vi "PicoScopeospaAdvancedTriggerPWQ.vi"(0 "handle in":i16=16384, 1 "Pulse Width Qualifier Settings":T3 {"Pulse Width Type" items=["None", "Less Than", "Greater Than", "In Range", "Out of Range"]}, 2 "Pulse Width Qualifier Trigger Properties":T1={"Channel A Trigger Properties"={"Threshold Mode"=0, "Available"=TRUE, "Direction"=2}, "Channel B Trigger Properties"={"Threshold Mode"=0, "Available"=FALSE, "Direction"=2}, "Channel C Trigger Properties"={"Threshold Mode"=0, "Available"=FALSE, "Direction"=2}, "Channel D Trigger Properties"={"Threshold Mode"=0, "Available"=FALSE, "Direction"=2}, "Channel E Trigger Properties"={"Threshold Mode"=0, "Available"=FALSE, "Direction"=2}, "Channel F Trigger Properties"={"Threshold Mode"=0, "Available"=FALSE, "Direction"=2}, "Channel G Trigger Properties"={"Threshold Mode"=0, "Available"=FALSE, "Direction"=2}, "Channel H Trigger Properties"={"Threshold Mode"=0, "Available"=FALSE, "Direction"=2}, "Port 0 Trigger Properties"={"Threshold Mode"=0, "Available"=FALSE, "Direction"=2}, "Port 1 Trigger Properties"={"Threshold Mode"=0, "Available"=FALSE, "Direction"=2}} {"Port 1 Trigger Properties"."Direction" items=["Rising"=2, "Falling"=3, "Rising Lower"=7, "Above"=0, "Below"=1, "Rising or Falling"=4, "Falling Lower"=8, "Below Lower"=6, "Above Lower"=5]; "Port 1 Trigger Properties"."Threshold Mode" items=["Level", "Window"]; "Port 0 Trigger Properties"."Direction" items=["Rising"=2, "Falling"=3, "Rising Lower"=7, "Above"=0, "Below"=1, "Rising or Falling"=4, "Falling Lower"=8, "Below Lower"=6, "Above Lower"=5]; "Port 0 Trigger Properties"."Threshold Mode" items=["Level", "Window"]; "Channel H Trigger Properties"."Direction" items=["Rising"=2, "Falling"=3, "Rising Lower"=7, "Above"=0, "Below"=1, "Rising or Falling"=4, "Falling Lower"=8, "Below Lower"=6, "Above Lower"=5]; "Channel H Trigger Properties"."Threshold Mode" items=["Level", "Window"]; "Channel G Trigger Properties"."Direction" items=["Rising"=2, "Falling"=3, "Rising Lower"=7, "Above"=0, "Below"=1, "Rising or Falling"=4, "Falling Lower"=8, "Below Lower"=6, "Above Lower"=5]; "Channel G Trigger Properties"."Threshold Mode" items=["Level", "Window"]; "Channel F Trigger Properties"."Direction" items=["Rising"=2, "Falling"=3, "Rising Lower"=7, "Above"=0, "Below"=1, "Rising or Falling"=4, "Falling Lower"=8, "Below Lower"=6, "Above Lower"=5]; "Channel F Trigger Properties"."Threshold Mode" items=["Level", "Window"]; "Channel E Trigger Properties"."Direction" items=["Rising"=2, "Falling"=3, "Rising Lower"=7, "Above"=0, "Below"=1, "Rising or Falling"=4, "Falling Lower"=8, "Below Lower"=6, "Above Lower"=5]; "Channel E Trigger Properties"."Threshold Mode" items=["Level", "Window"]; "Channel D Trigger Properties"."Direction" items=["Rising"=2, "Falling"=3, "Rising Lower"=7, "Above"=0, "Below"=1, "Rising or Falling"=4, "Falling Lower"=8, "Below Lower"=6, "Above Lower"=5]; "Channel D Trigger Properties"."Threshold Mode" items=["Level", "Window"]; "Channel C Trigger Properties"."Direction" items=["Rising"=2, "Falling"=3, "Rising Lower"=7, "Above"=0, "Below"=1, "Rising or Falling"=4, "Falling Lower"=8, "Below Lower"=6, "Above Lower"=5]; "Channel C Trigger Properties"."Threshold Mode" items=["Level", "Window"]; "Channel B Trigger Properties"."Direction" items=["Rising"=2, "Falling"=3, "Rising Lower"=7, "Above"=0, "Below"=1, "Rising or Falling"=4, "Falling Lower"=8, "Below Lower"=6, "Above Lower"=5]; "Channel B Trigger Properties"."Threshold Mode" items=["Level", "Window"]; "Channel A Trigger Properties"."Direction" items=["Rising"=2, "Falling"=3, "Rising Lower"=7, "Above"=0, "Below"=1, "Rising or Falling"=4, "Falling Lower"=8, "Below Lower"=6, "Above Lower"=5]; "Channel A Trigger Properties"."Threshold Mode" items=["Level", "Window"]}, 11 "error in":errorcluster, 13 "Pulse Width Qualifier Conditions":T2 {"Port 1" items=["Don't Care", "True", "False"]; "Channel H" items=["Don't Care", "True", "False"]; "Channel G" items=["Don't Care", "True", "False"]; "Channel F" items=["Don't Care", "True", "False"]; "Channel E" items=["Don't Care", "True", "False"]; "Aux" items=["Don't Care", "True", "False"]; "Port 0" items=["Don't Care", "True", "False"]; "Channel D" items=["Don't Care", "True", "False"]; "Channel C" items=["Don't Care", "True", "False"]; "Channel B" items=["Don't Care", "True", "False"]; "Channel A" items=["Don't Care", "True", "False"]; "Condition Logic" items=["AND", "OR", "XOR"]}) -> (4 "handle out":i16=16384, 15 "error out":errorcluster)   [LabVIEW 2010]
doc: "This sub VI is an interface for the advanced trigger features of the oscilloscope to support Pulse width qualifier (PWQ)."
uses:
  ps6000a.dll
  psospa.dll
panel:
  in  "PWQ Info Action XOR":bool=TRUE
  in  "PWQ Info Action OR":bool=TRUE
  # "For Condition Logic Suggested settings;\nFor AND, XOR logic-(parallel triggers)\nUse level-type triggers (Level or Inside/outside Window Triggers)\n\nFor OR logic- (single channel)\nUse edge types (e.g. rising, falling, entering window)"
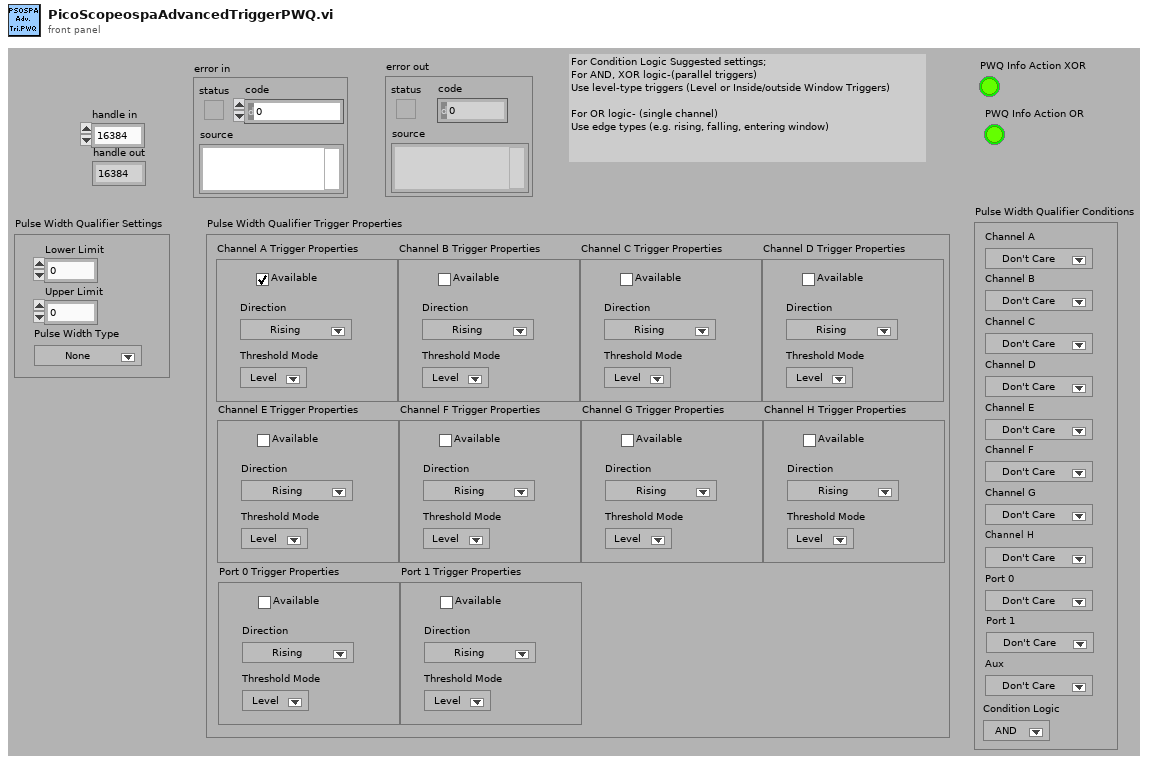
[diagram p1: front panel]
types:
  T1 = cluster{"Channel A Trigger Properties":cluster{"Threshold Mode":i32, "Available":bool, "Direction":u32}, "Channel B Trigger Properties":cluster{"Threshold Mode":i32, "Available":bool, "Direction":u32}, "Channel C Trigger Properties":cluster{"Threshold Mode":i32, "Available":bool, "Direction":u32}, "Channel D Trigger Properties":cluster{"Threshold Mode":i32, "Available":bool, "Direction":u32}, "Channel E Trigger Properties":cluster{"Threshold Mode":i32, "Available":bool, "Direction":u32}, "Channel F Trigger Properties":cluster{"Threshold Mode":i32, "Available":bool, "Direction":u32}, "Channel G Trigger Properties":cluster{"Threshold Mode":i32, "Available":bool, "Direction":u32}, "Channel H Trigger Properties":cluster{"Threshold Mode":i32, "Available":bool, "Direction":u32}, "Port 0 Trigger Properties":cluster{"Threshold Mode":i32, "Available":bool, "Direction":u32}, "Port 1 Trigger Properties":cluster{"Threshold Mode":i32, "Available":bool, "Direction":u32}}
  T2 = cluster{"Channel A":u16, "Channel B":u16, "Channel C":u16, "Channel D":u16, "Channel E":u16, "Channel F":u16, "Channel G":u16, "Channel H":u16, "Port 0":u16, "Port 1":u16, "Aux":u16, "Condition Logic":u16}
  T3 = cluster{"Lower Limit":u32, "Upper Limit":u32, "Pulse Width Type":u32}
  T4 = cluster{"Threshold Mode":i32, "Available":bool, "Direction":u32}[]
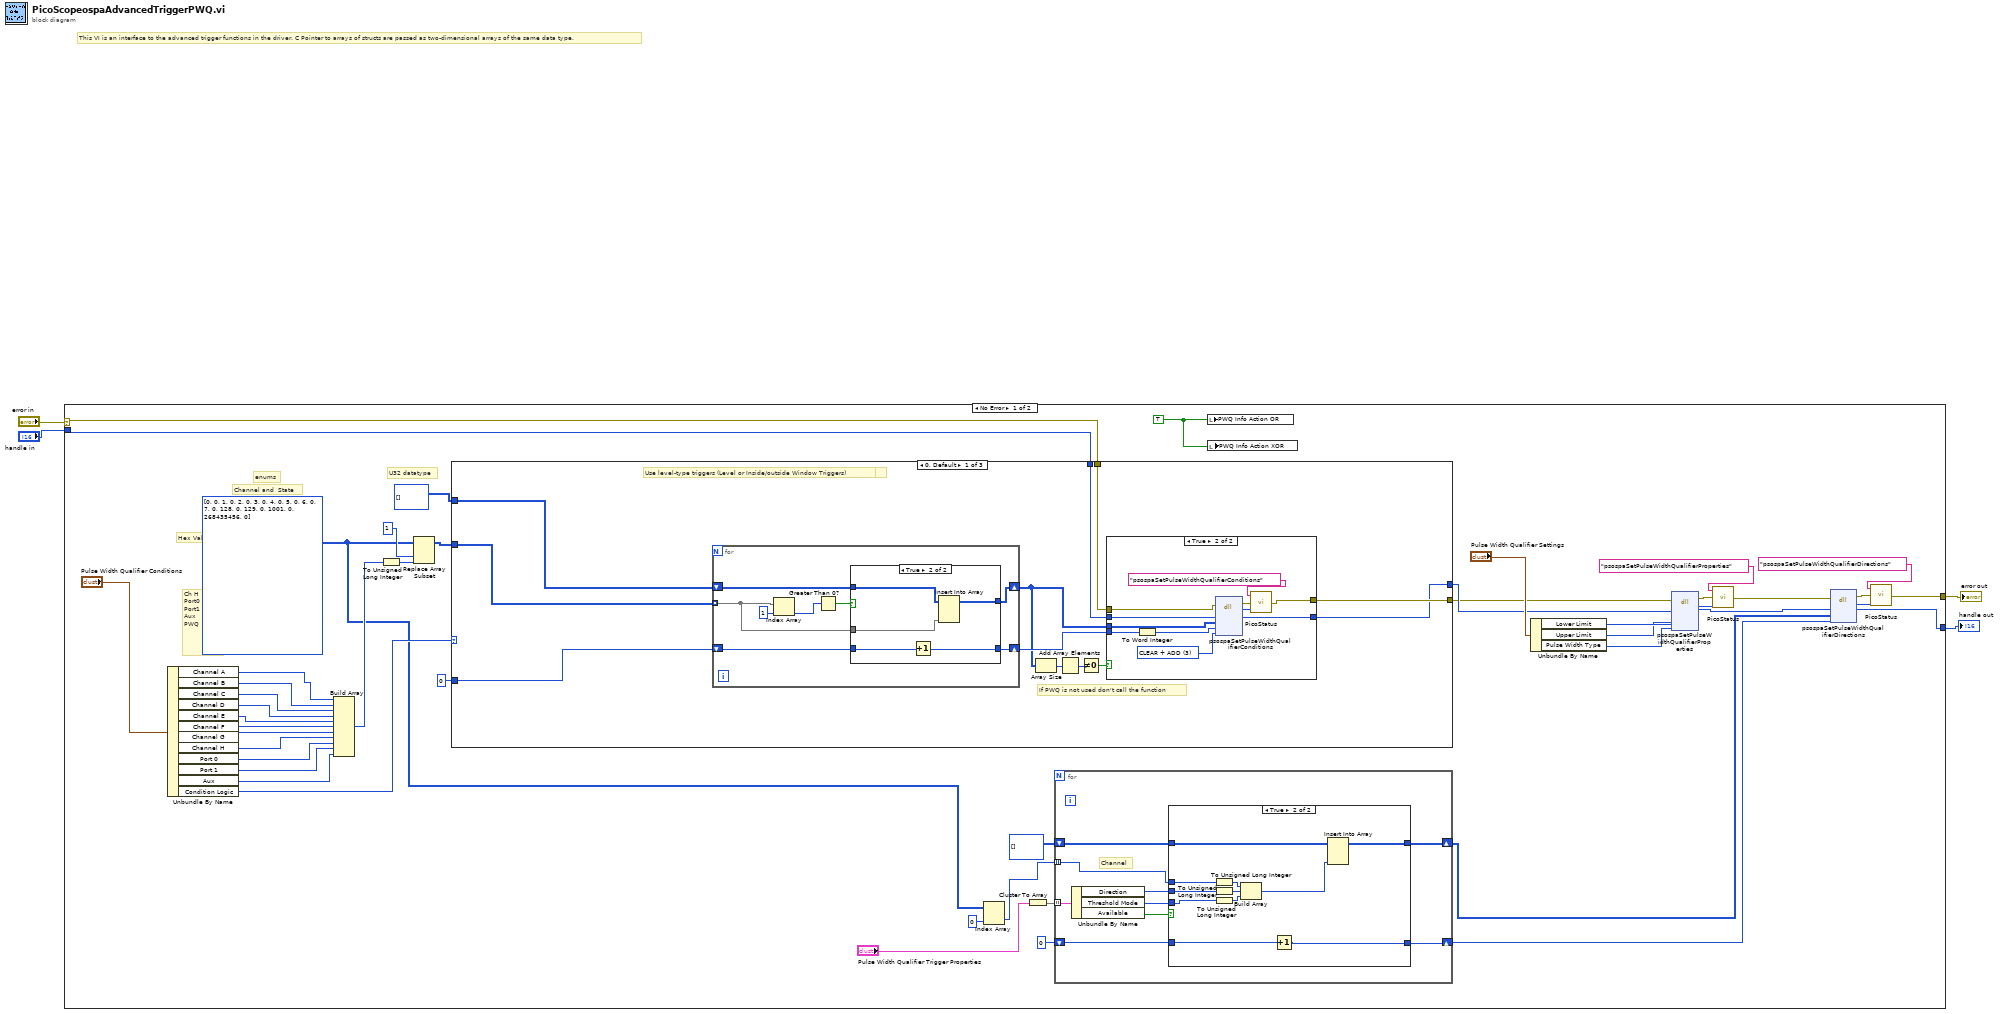
[diagram p0: block diagram]
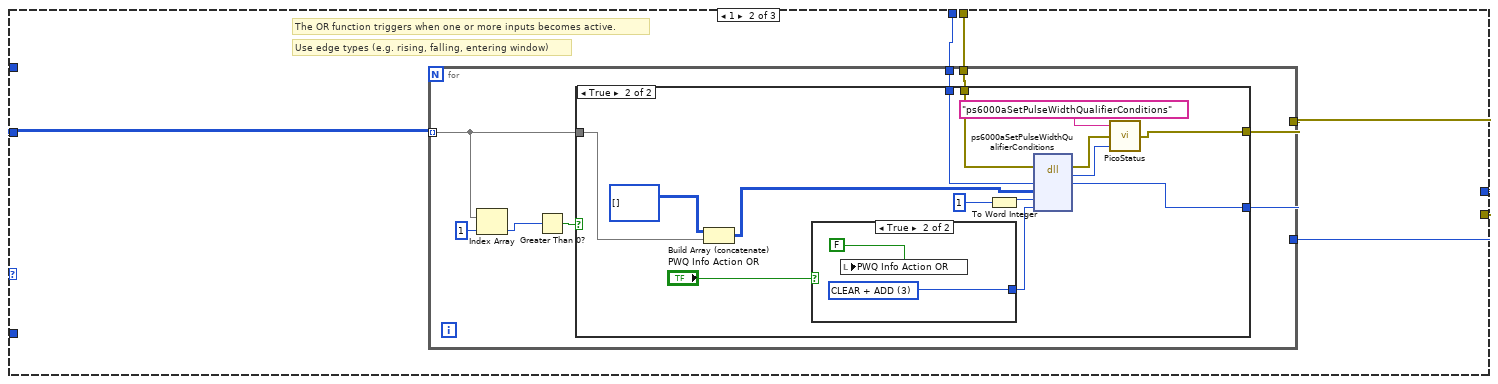
[diagram p5: hidden frame]
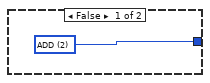
[diagram p7: hidden frame]
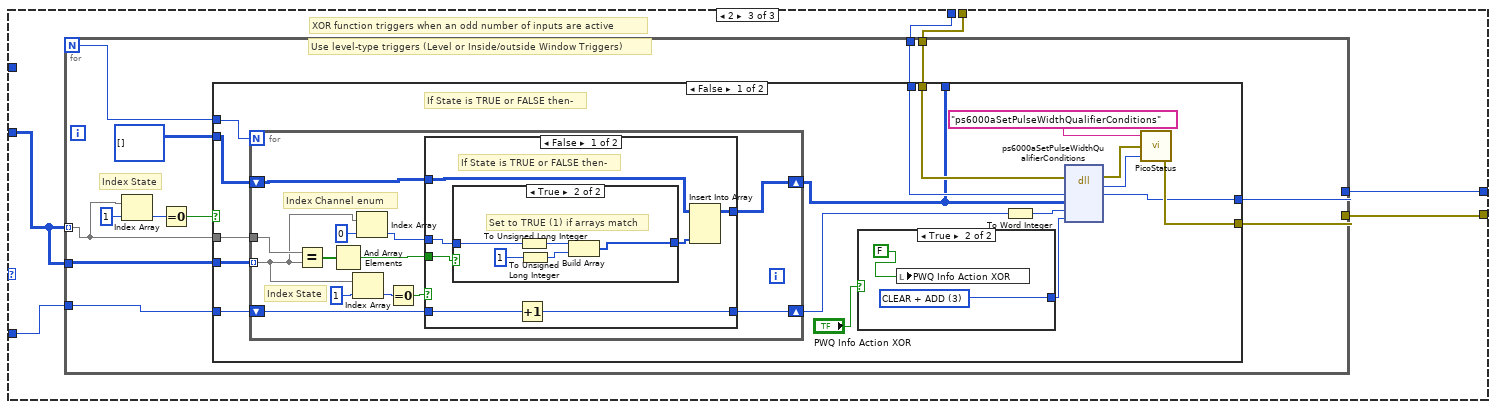
[diagram p8: hidden frame]
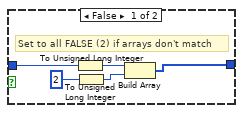
[diagram p9: hidden frame]
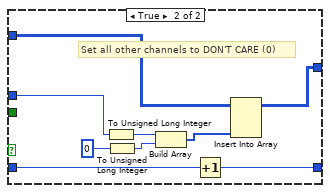
[diagram p10: hidden frame]
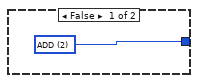
[diagram p11: hidden frame]
diagram:
  # "This VI is an interface to the advanced trigger functions in the driver. C Pointer to arrays of structs are passed as two-dimensional arrays of the same data type."
  n1 = case shown="No Error" "error in" {
    selector: "error in" -> [w6 w226]
    tunnel: "handle in" -> [w5 w227]
    tunnel: [w7 w227] -> w2
    tunnel: [w8 w226] -> w1
    frame No Error {
      w26 = TRUE ("PWQ Info Action XOR")
      w9 = u32[][] [[0, 0], [1, 0], [2, 0], [3, 0], [4, 0], [5, 0], [6, 0], [7, 0], [128, 0], [129, 0], [1001, 0], [268435456, 0]]
      # "U32 datatype"
      # "enums"
      # "Ch H\nPort0\nPort1\nAux\nPWQ"
      # "Channel and  State"
      # "Hex Values"
      n2 = Unbundle By Name("Pulse Width Qualifier Conditions") -> ("Channel A"=w36:u16, "Channel B"=w35:u16, "Channel C"=w34:u16, "Channel D"=w33:u16, "Channel E"=w32:u16, "Channel F"=w31:u16, "Channel G"=w30:u16, "Channel H"=w29:u16, "Port 0"=w28:u16, "Port 1"=w27:u16, "Aux"=w10:u16, "Condition Logic"=w11:u16)
      n3 = Build Array(w36, w35, w34, w33, w32, w31, w30, w29, w28, w27, w10) -> (w50:u16[])
      n4 = To Unsigned Long Integer(number=w50) -> (unsigned 32bit integer=w39:u32[])
      n5 = Replace Array Subset(array=w9, new element=w39, index (col)=1 ("disabled index (col)")) -> (w38:u32[][])  [unwired: 1 in]
      n6 = case shown="0, Default" w11 {
        tunnel: u32[][] [] -> [w85 _ _]
        tunnel: i16 0 -> [w84 _ w146]
        tunnel: w6 -> [w81 w118 w151]
        tunnel: w5 -> [w80 w117 w150]
        tunnel: [w79 w116 w149] -> w40
        tunnel: [w78 w115 w148] -> w41
        tunnel: w38 -> [w82 w114 w147]
        frame 0, Default {
          # "If PWQ is not used don't call the function"
          # "AND function requires both inputs to be active before it will trigger."
          # "Use level-type triggers (Level or Inside/outside Window Triggers)"
          n7 = for {
            shift-right: [w105] -> w83
            shift-left: w84 -> [w104]
            shift-right: [w103] -> w77
            shift-left: w85 -> [w106]
            tunnel: w82 -> [w101] mode=indexing
            n8 = Index Array(array=w101, index=1) -> (element=w100:u32)
            n9 = Greater Than 0?(x=w100) -> (x > 0?=w102:bool)
            n10 = case shown="True" w102 {
              tunnel: w106 -> [w108 w113]
              tunnel: [w108 w112] -> w103
              tunnel: [w107 w111] -> w105
              tunnel: w104 -> [w107 w110]
              tunnel: w101 -> [_ w109]
              frame False {
              }
              frame True {
                n11 = Increment(x=w110) -> (x+1=w111:i16)
                n12 = Insert Into Array(array=w113, new element=w109) -> (w112:u32[][])  [unwired: 2 in]
              }
            }
          }
          n13 = Array Size(array=w77) -> (size(s)=w75:i32[])
          n14 = Add Array Elements(numeric array=w75) -> (sum=w76:i32)
          n15 = Not Equal To 0?(x=w76) -> (x != 0?=w74:bool)
          n16 = case shown="True" w74 {
            tunnel: w83 -> [_ w98]
            tunnel: w81 -> [w87 w94]
            tunnel: w80 -> [w86 w93]
            tunnel: w77 -> [_ w90]
            tunnel: [w87 w89] -> w79
            tunnel: [w86 w88] -> w78
            frame False {
            }
            frame True {
              w92 = u32 3 items=["CLEAR + ADD"=3, "CLEAR"=1, "ADD"=2] ("Condition Action")
              n17 = To Word Integer(number=w98) -> (16bit integer=w91:i16)
              n18 = dll-call lib="psospa.dll" fn="psospaSetPulseWidthQualifierConditions" ("ps3000.dll:_ps3000_open_unit@0")(error in=w94, "handle"=w93, "conditions"=w90, "nConditions"=w91, "action"=w92) -> (error out=w97:errorcluster, "PICO_STATUS"=w96:u32, "handle"=w88:i16)  [unwired: 5 in, 1 out]
              n19 = call "PicoStatus.vi"("PICO STATUS"=w96, "error in"=w97, "source"="psospaSetPulseWidthQualifierConditions") -> ("error out"=w89:errorcluster)
            }
          }
        }
        frame 1 {
          # "Use edge types (e.g. rising, falling, entering window)"
          # "The OR function triggers when one or more inputs becomes active."
          n20 = for {
            tunnel: w118 -> [w126]
            tunnel: w117 -> [w125]
            tunnel: [w124] -> w116
            tunnel: [w123] -> w115
            tunnel: w114 -> [w121] mode=indexing
            n21 = Index Array(array=w121, index=1) -> (element=w120:u32)
            n22 = Greater Than 0?(x=w120) -> (x > 0?=w119:bool)
            n23 = case shown="True" w119 {
              tunnel: w126 -> [w127 w138]
              tunnel: w125 -> [w128 w137]
              tunnel: [w127 w135] -> w124
              tunnel: [w128 w134] -> w123
              tunnel: w121 -> [_ w129]
              frame False {
              }
              frame True {
                n24 = Build Array (concatenate)(u32[][] [], w129) -> (w131:u32[][])
                n25 = case shown="True" "PWQ Info Action OR" {
                  tunnel: [w143 w145] -> w136
                  frame False {
                    w143 = u32 2 items=["CLEAR"=1, "ADD"=2, "CLEAR + ADD"=3] ("Condition Action")
                  }
                  frame True {
                    w145 = u32 3 items=["CLEAR"=1, "ADD"=2, "CLEAR + ADD"=3] ("Condition Action")
                    n26 = local write "PWQ Info Action OR"(FALSE ("Boolean")) -> ()
                  }
                }
                n27 = To Word Integer(number=i16 1) -> (16bit integer=w142:i16)
                n28 = dll-call lib="ps6000a.dll" fn="ps6000aSetPulseWidthQualifierConditions" ("ps3000.dll:_ps3000_open_unit@0")(error in=w138, "handle"=w137, "conditions"=w131, "nConditions"=w142, "action"=w136) -> (error out=w141:errorcluster, "PICO_STATUS"=w140:u32, "handle"=w134:i16)  [unwired: 5 in, 1 out]
                n29 = call "PicoStatus.vi"("PICO STATUS"=w140, "error in"=w141, "source"="ps6000aSetPulseWidthQualifierConditions") -> ("error out"=w135:errorcluster)
              }
            }
          }
        }
        frame 2 {
          # "Use level-type triggers (Level or Inside/outside Window Triggers)"
          # "XOR function triggers when an odd number of inputs are active"
          n30 = for {
            N -> [w159]
            tunnel: w151 -> [w163]
            tunnel: w150 -> [w162]
            tunnel: [w161] -> w149
            tunnel: [w160] -> w148
            tunnel: w147 -> [w153] mode=indexing
            tunnel: w147 -> [w156]
            tunnel: w146 -> [w157]
            # "Index State"
            n31 = Index Array(array=w153, index=1) -> (element=w154:u32)
            n32 = Equal To 0?(x=w154) -> (x = 0?=w152:bool)
            n33 = case shown="False" w152 {
              tunnel: w163 -> [w180 w223]
              tunnel: w162 -> [w179 w224]
              tunnel: [w178 w223] -> w161
              tunnel: [w177 w224] -> w160
              tunnel: [w175 w225] -> _
              tunnel: w159 -> [w174 _]
              tunnel: u32[][] [] -> [w173 w225]
              tunnel: w157 -> [w172 _]
              tunnel: w156 -> [w171 _]
              tunnel: w153 -> [w170 _]
              frame False {
                # "If State is TRUE or FALSE then-"
                n34 = for {
                  N: w174 -> [_]
                  shift-right: [w192] -> w176
                  shift-left: w172 -> [w193]
                  shift-right: [w181] -> w175
                  shift-left: w173 -> [w182]
                  tunnel: w170 -> [w189]
                  tunnel: w171 -> [w185] mode=indexing
                  # "Index State"
                  # "Index Channel enum"
                  n35 = Equal?(x=w189, y=w185) -> (x = y?=w183:bool[])
                  n36 = And Array Elements(Boolean array=w183) -> (logical AND=w188:bool)
                  n37 = Index Array(array=w185, index=1) -> (element=w186:u32)
                  n38 = Index Array(array=w185, index=0) -> (element=w190:u32)
                  n39 = Equal To 0?(x=w186) -> (x = 0?=w184:bool)
                  n40 = case shown="False" w184 {
                    tunnel: w193 -> [w200 w211]
                    tunnel: [w199 w212] -> w192
                    tunnel: w190 -> [w198 w215]
                    tunnel: w188 -> [w197 _]
                    tunnel: w182 -> [w196 w214]
                    tunnel: [w194 w213] -> w181
                    frame False {
                      # "If State is TRUE or FALSE then-"
                      n41 = case shown="True" w197 {
                        tunnel: [w205 w210] -> w195
                        tunnel: w198 -> [w204 w209]
                        frame False {
                          # "Set to all FALSE (2) if arrays don't match"
                          n42 = To Unsigned Long Integer(number=w204) -> (unsigned 32bit integer=w202:u32)
                          n43 = To Unsigned Long Integer(number=u32 2) -> (unsigned 32bit integer=w203:u32)
                          n44 = Build Array(w202, w203) -> (w205:u32[])
                        }
                        frame True {
                          # "Set to TRUE (1) if arrays match"
                          n45 = To Unsigned Long Integer(number=w209) -> (unsigned 32bit integer=w207:u32)
                          n46 = To Unsigned Long Integer(number=u32 1) -> (unsigned 32bit integer=w208:u32)
                          n47 = Build Array(w207, w208) -> (w210:u32[])
                        }
                      }
                      n48 = Increment(x=w200) -> (x+1=w199:i16)
                      n49 = Insert Into Array(array=w196, new element=w195) -> (w194:u32[][])  [unwired: 2 in]
                    }
                    frame True {
                      # "Set all other channels to DON'T CARE (0)"
                      n50 = To Unsigned Long Integer(number=w215) -> (unsigned 32bit integer=w217:u32)
                      n51 = To Unsigned Long Integer(number=u32 0) -> (unsigned 32bit integer=w218:u32)
                      n52 = Build Array(w217, w218) -> (w219:u32[])
                      n53 = Increment(x=w211) -> (x+1=w212:i16)
                      n54 = Insert Into Array(array=w214, new element=w219) -> (w213:u32[][])  [unwired: 2 in]
                    }
                  }
                }
                n55 = case shown="True" "PWQ Info Action XOR" {
                  tunnel: [w220 w222] -> w164
                  frame False {
                    w220 = u32 2 items=["CLEAR + ADD"=3, "CLEAR"=1, "ADD"=2] ("Condition Action")
                  }
                  frame True {
                    w222 = u32 3 items=["CLEAR + ADD"=3, "CLEAR"=1, "ADD"=2] ("Condition Action")
                    n56 = local write "PWQ Info Action XOR"(FALSE ("Boolean")) -> ()
                  }
                }
                n57 = To Word Integer(number=w176) -> (16bit integer=w169:i16)
                n58 = dll-call lib="ps6000a.dll" fn="ps6000aSetPulseWidthQualifierConditions" ("ps3000.dll:_ps3000_open_unit@0")(error in=w180, "handle"=w179, "conditions"=w175, "nConditions"=w169, "action"=w164) -> (error out=w168:errorcluster, "PICO_STATUS"=w167:u32, "handle"=w177:i16)  [unwired: 5 in, 1 out]
                n59 = call "PicoStatus.vi"("PICO STATUS"=w167, "error in"=w168, "source"="ps6000aSetPulseWidthQualifierConditions") -> ("error out"=w178:errorcluster)
              }
              frame True {
              }
            }
          }
        }
      }
      n60 = Index Array(array=w9, index (col)=0 ("disabled index (col)")) -> (element=w12:u32[])  [unwired: 1 in]
      n61 = Cluster To Array(cluster="Pulse Width Qualifier Trigger Properties") -> (array=w18:T4)
      n62 = for {
        tunnel: w18 -> [w60] mode=indexing
        shift-right: [w55] -> w16
        shift-left: u32[][] [] -> [w56]
        shift-right: [w53] -> w14
        shift-left: i16 0 ("nDirections") -> [w54]
        tunnel: w12 -> [w52] mode=indexing
        # "Channel"
        n63 = Unbundle By Name(w60) -> ("Direction"=w58:u32, "Threshold Mode"=w57:i32, "Available"=w59:bool)
        n64 = case shown="True" w59 {
          tunnel: w52 -> [_ w69]
          tunnel: w58 -> [_ w68]
          tunnel: w57 -> [_ w67]
          tunnel: w56 -> [w62 w66]
          tunnel: [w62 w65] -> w55
          tunnel: [w61 w64] -> w53
          tunnel: w54 -> [w61 w63]
          frame False {
          }
          frame True {
            n65 = To Unsigned Long Integer(number=w69) -> (unsigned 32bit integer=w71:u32)
            n66 = To Unsigned Long Integer(number=w68) -> (unsigned 32bit integer=w72:u32)
            n67 = To Unsigned Long Integer(number=w67) -> (unsigned 32bit integer=w70:u32)
            n68 = Build Array(w71, w72, w70) -> (w73:u32[])
            n69 = Increment(x=w63) -> (x+1=w64:i16)
            n70 = Insert Into Array(array=w66, new element=w73) -> (w65:u32[][])  [unwired: 2 in]
          }
        }
      }
      n71 = local write "PWQ Info Action OR"(w26) -> ()
      n72 = local write "PWQ Info Action XOR"(w26) -> ()
      n73 = Unbundle By Name("Pulse Width Qualifier Settings") -> ("Lower Limit"=w47:u32, "Upper Limit"=w46:u32, "Pulse Width Type"=w45:u32)
      n74 = dll-call lib="psospa.dll" fn="psospaSetPulseWidthQualifierProperties" ("ps3000.dll:_ps3000_open_unit@0")(error in=w40, "handle"=w41, "lower"=w47, "upper"=w46, "type"=w45) -> (error out=w49:errorcluster, "PICO_STATUS"=w44:u32, "handle"=w21:i16)  [unwired: 5 in, 1 out]
      n75 = call "PicoStatus.vi"("PICO STATUS"=w44, "error in"=w49, "source"="psospaSetPulseWidthQualifierProperties") -> ("error out"=w22:errorcluster)
      n76 = dll-call lib="psospa.dll" fn="psospaSetPulseWidthQualifierDirections" ("ps3000.dll:_ps3000_open_unit@0")(error in=w22, "handle"=w21, "directions"=w16, "nDirections"=w14) -> (error out=w25:errorcluster, "PICO_STATUS"=w24:u32, "handle"=w7:i16)  [unwired: 4 in, 1 out]
      n77 = call "PicoStatus.vi"("PICO STATUS"=w24, "error in"=w25, "source"="psospaSetPulseWidthQualifierDirections") -> ("error out"=w8:errorcluster)
    }
    frame Error {
    }
  }
  "handle out" <- w2
  "error out" <- w1
